vi "AutoDrive_sub.vi"(8 "EncoderVals":i32[](array[numeric]), 9 "Target Heading (Degrees)":i16, 10 "Drive Control":T2={"Left X"=0, "Left Y"=0, "Right X"=0, "Power (100)"=100, "Wait (ms)"=100, "Enc/Deg Target"=0, "Move Type"=enum."Wait"} {"Power (100)" min=-100 max=100}, 11 "NXT/EV3":T1) -> (0 "EncoderVals":i32[](array[numeric]), 3 "NXT/EV3 out":T1)   [LabVIEW 2012, in "Mecanum Drive.lvrbt"]
uses:
  Mecanum Drive.lvrbt
  SubVIs/auto_drive_TYP.ctl
  <vilib>/NXT/Subs/LVHSConnector.ctl
  <vilib>/NXT/LegoClasses/BrickReference/BrickReference.lvclass
  <vilib>/FTC/FTC ControllerState.ctl
  <vilib>/FTC/FTC POVState.ctl
  <vilib>/NXT/Hardware/Plugins/Tetrix DC Motor/TetrixDCMotorAddress.ctl
  <vilib>/NXT/HiTechnic/HiTechnic Controls/HiTechnic Port.ctl
  <vilib>/NXT/Block Support/NXT_InputPort.ctl
  <vilib>/NXT/NXTIO Xnodes/NXTIONodeSubVIs/TETRIX IO Move DC Motors.vi
  <vilib>/NXT/Dual Mode Library/Waits/Wait_Num(msec).vi
  <vilib>/NXT/NXTIO Xnodes/NXTIONodeSubVIs/TETRIX IO Motor Status.vi
  <vilib>/NXT/Dual Mode Library/Display/drawNumber.vi
  <vilib>/NXT/NXTIO Xnodes/AddressXNode/NXTIOAddress.xnode
  <vilib>/NXT/NXTIO Xnodes/NXTIOXNode/NXTIO.xnode
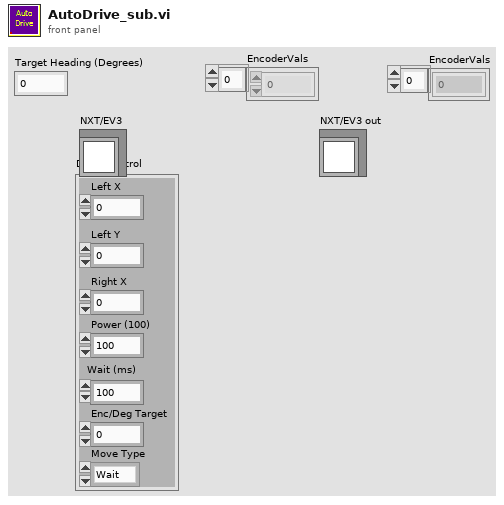
[diagram p1: front panel]
types:
  T1 = typedef "LVHSConnector.ctl" = refnum<class "BrickReference.lvclass">
  T2 = typedef "auto_drive_TYP.ctl" = cluster{"Left X":i8, "Left Y":i8, "Right X":i8, "Power (100)":i8, "Wait (ms)":u32, "Enc/Deg Target":i32, "Move Type":enum16{"Relative Degrees", "Wait", "Encoder"}}
  T3 = typedef "FTC ControllerState.ctl" = cluster{"Left X":i8, "Left Y":i8, "Right X":i8, "Right Y":i8, "Button Encoding 9-12":u8, "Button Encoding 1-8":u8, "POV":T4}
  T4 = typedef "FTC POVState.ctl" = i8
  T5 = typedef "TetrixDCMotorAddress.ctl" = i32
  T6 = typedef "HiTechnic Port.ctl" = cluster{"Port":T7, "MUX Port":u8}
  T7 = typedef "NXT_InputPort.ctl" = u32
  T8 = cluster{"TetrixDCMotor":T5, "TetrixDCMotor 2":T5}
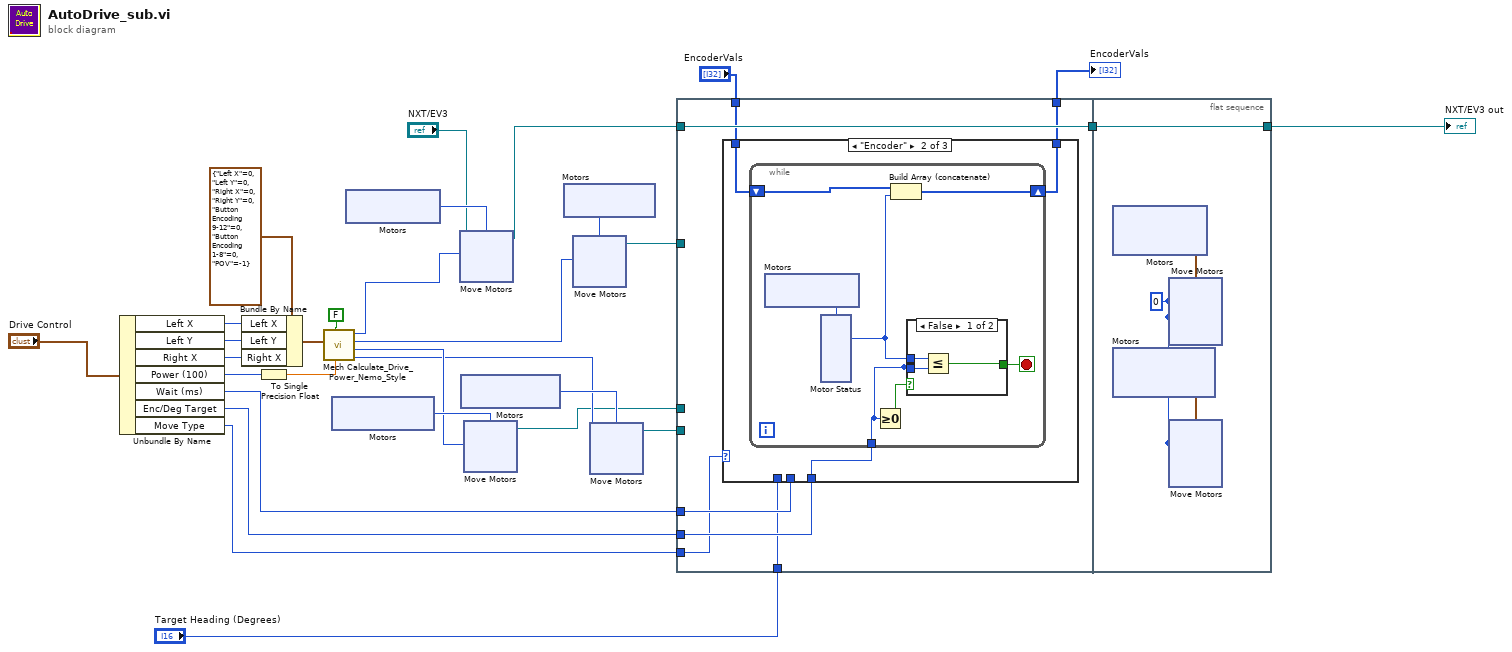
[diagram p0: block diagram]
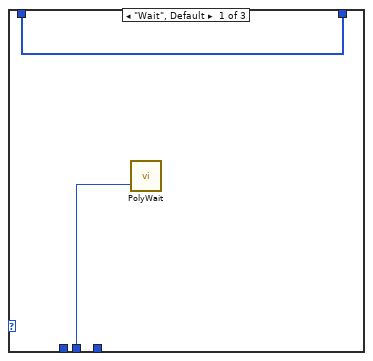
[diagram p2: hidden frame]
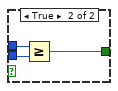
[diagram p3: hidden frame]
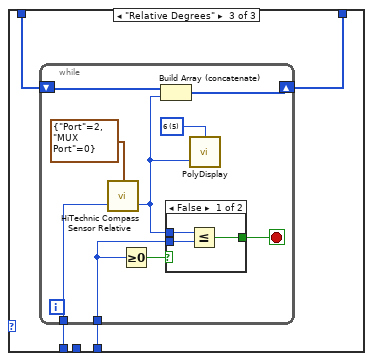
[diagram p4: hidden frame]
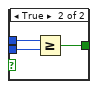
[diagram p5: hidden frame]
diagram:
  n1 = Unbundle By Name("Drive Control") -> ("Left X"=w17:i8, "Left Y"=w16:i8, "Right X"=w15:i8, "Power (100)"=w9:i8, "Wait (ms)"=w10:u32, "Enc/Deg Target"=w5:i32, "Move Type"=w4:enum16{"Relative Degrees", "Wait", "Encoder"})
  n2 = Bundle By Name(cluster=T3 {"Left X"=0, "Left Y"=0, "Right X"=0, "Right Y"=0, "Button Encoding 9-12"=0, "Button Encoding 1-8"=0, "POV"=-1} ("Controller State"), "Left X"=w17, "Left Y"=w16, "Right X"=w15) -> (w21:T3)
  n3 = To Single Precision Float(number=w9) -> (single precision float=w8:sgl)
  n4 = call "Mech Calculate_Drive_Power_Nemo_Style.vi"("Power"=w8, "Reverse"=FALSE, "Controller State"=w21) -> ("Right Rear Power"=w23:i8, "Right Front Power"=w24:i8, "Left Rear Power"=w25:i8, "Left Front Power"=w22:i8)  [unwired: 5 in]
  n5 = xnode ("Motors")() -> ("Motor"=w30:T5)
  n6 = xnode ("Motors")() -> ("Motor"=w27:T5)
  n7 = xnode ("Move Motors")("Power/Speed 1"=w22, "Motors"=w27, "NXT/EV3"="NXT/EV3") -> ("NXT/EV3"=w14:T1)
  n8 = xnode ("Motors")() -> ("Motor"=w29:T5)
  n9 = xnode ("Move Motors")("Power/Speed 1"=w24, "Motors"=w30) -> ("NXT/EV3"=w11:T1)  [unwired: 1 in]
  n10 = xnode ("Motors")() -> ("Motor"=w28:T5)
  n11 = xnode ("Move Motors")("Power/Speed 1"=w25, "Motors"=w28) -> ("NXT/EV3"=w13:T1)  [unwired: 1 in]
  n12 = xnode ("Move Motors")("Power/Speed 1"=w23, "Motors"=w29) -> ("NXT/EV3"=w12:T1)  [unwired: 1 in]
  n13 = flat-sequence {
    tunnel: w14 -> [w37]
    tunnel: w13 -> [_]
    tunnel: w12 -> [_]
    tunnel: w11 -> [_]
    tunnel: w10 -> [w36]
    tunnel: [w37] -> w6
    tunnel: w5 -> [w35]
    tunnel: w4 -> [w34]
    tunnel: "Target Heading (Degrees)" -> [w33]
    tunnel: "EncoderVals" -> [w32]
    tunnel: [w31] -> w1
    tunnel: [w87] -> w7
    tunnel: w6 -> [w87]
    frame #0 {
      n14 = case shown="\"Encoder\"" w34 {
        tunnel: w36 -> [w39 _ _]
        tunnel: w35 -> [_ w42 w67]
        tunnel: w33 -> [_ _ w68]
        tunnel: w32 -> [w38 w41 w66]
        tunnel: [w38 w40 w65] -> w31
        frame "Wait", Default {
          n15 = call-poly <vilib>:"PolyWait.vi"("Time (100 msec)"=w39) -> ()  [unwired: 3 in, 1 out]
        }
        frame "Encoder" {
          n16 = while {
            tunnel: w42 -> [w43]
            shift-right: [w48] -> w40
            shift-left: w41 -> [w47]
            stop <- w44 stop-if-true
            n17 = xnode "Motors"() -> ("Motor"=w49:T5)
            n18 = xnode "Motor Status"("Motors"=w49) -> ("Position 1"=w45:i32)  [unwired: 1 in, 2 out]
            n19 = Greater Or Equal To 0?(x=w43) -> (x >= 0?=w46:bool)
            n20 = Build Array (concatenate)(w47, w45) -> (w48:i32[])
            n21 = case shown="False" w46 {
              tunnel: w43 -> [_ w54]
              tunnel: w45 -> [w52 w55]
              tunnel: [w50 w53] -> w44
              tunnel: w43 -> [w51 _]
              frame False {
                n22 = Less Or Equal?(x=w52, y=w51) -> (x <= y?=w50:bool)
              }
              frame True {
                n23 = Greater Or Equal?(x=w55, y=w54) -> (x >= y?=w53:bool)
              }
            }
          }
        }
        frame "Relative Degrees" {
          n24 = while {
            tunnel: w68 -> [w76]
            tunnel: w67 -> [w73]
            shift-right: [w71] -> w65
            shift-left: w66 -> [w69]
            stop <- w75 stop-if-true
            w74 = i16 5 items=["1", "2", "3", "4", "5", "6", "7", "8", "9", "10", "11", "12"] ("Line")
            n25 = call <vilib>:"HiTechnic Compass Sensor Relative.vi"("Target Heading (Degrees)"=w76, "Port/MUX"=T6 {"Port"=2, "MUX Port"=0}) -> ("Relative Heading (Degrees)"=w70:i32)  [unwired: 1 in, 1 out]
            n26 = Greater Or Equal To 0?(x=w73) -> (x >= 0?=w72:bool)
            n27 = Build Array (concatenate)(w69, w70) -> (w71:i32[])
            n28 = case shown="False" w72 {
              tunnel: w73 -> [w78 w83]
              tunnel: [w80 w82] -> w75
              tunnel: w70 -> [w79 w81]
              frame False {
                n29 = Less Or Equal?(x=w79, y=w78) -> (x <= y?=w80:bool)
              }
              frame True {
                n30 = Greater Or Equal?(x=w81, y=w83) -> (x >= y?=w82:bool)
              }
            }
            n31 = call-poly <vilib>:"PolyDisplay.vi"("number"=w70, "Line"=w74) -> ()  [unwired: 2 in, 1 out]
          }
        }
      }
    }
    frame #1 {
      w84 = i8 0 ("Power/Speed 1")
      n32 = xnode "Motors"() -> ("Motor"=w86:cluster{"TetrixDCMotor":T5, "TetrixDCMotor":T5})
      n33 = xnode "Motors"() -> ("Motor"=w85:cluster{"TetrixDCMotor":T5, "TetrixDCMotor":T5})
      n34 = xnode "Move Motors"("Power/Speed 2"=w84, "Power/Speed 1"=w84, "Motors"=w86) -> ()  [unwired: 1 in, 1 out]
      n35 = xnode "Move Motors"("Power/Speed 2"=w84, "Power/Speed 1"=w84, "Motors"=w85) -> ()  [unwired: 1 in, 1 out]
    }
  }
  "NXT/EV3 out" <- w7
  "EncoderVals" <- w1
